vi "Interface.vi"() -> ()   [LabVIEW 2016, in "Operation Interface.lvclass"]
uses:
  Operation Interface.lvclass
  Robot/Universal Robot/Universal Robot.lvclass
  C:/_Code/Development/URLabVIEWInterface/Classes/Application/Application Interfaces/Application Interface/Application Interface.lvclass
  Operation Interface.lvclass/Operation Interface.ctl
  Application Interface/FGVAction.ctl
  Application.lvclass
  Application Interface/Application Interface.lvclass
panel:
  out "Robot Mode":string
  out "robotModeColor":u32(colorbox)
  out "Operational Mode":string
  in  "powerOn":bool
  in  "brakeRelease":bool
  out "Safety Status":string
  out "safetyStatusColor":u32(colorbox)
  in  "restartSafety":bool
  in  "unlockProtectiveStop":bool
  in  "shutdownRobot":bool
  in  "sample rate (ms)":i32
  in  "interface":refnum<class "Operation Interface.lvclass">
  in  "robot":refnum<class "Universal Robot.lvclass">
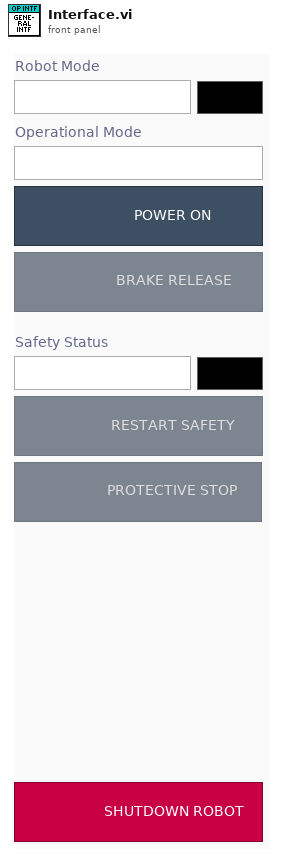
[diagram p1: front panel]
types:
  T1 = typedef "Universal Robot.lvclass/RobotStatus.ctl" = cluster{"Robot Mode":T2, "Operational Mode":T3, "Safety Status":T4, "Remote Control":bool}
  T2 = typedef "Universal Robot.lvclass/RobotMode.ctl" = enum16{"INVALID", "NO_CONTROLLER", "DISCONNECTED", "CONFIRM_SAFETY", "BOOTING", "POWER_OFF", "POWER_ON", "IDLE", "BACKDRIVE", "RUNNING"}
  T3 = typedef "Universal Robot.lvclass/OperationalMode.ctl" = enum16{"NONE", "MANUAL", "AUTOMATIC"}
  T4 = typedef "Universal Robot.lvclass/SafetyStatus.ctl" = enum16{"INVALID", "NORMAL", "REDUCED", "PROTECTIVE_STOP", "RECOVERY", "SAFEGUARD_STOP", "SYSTEM_EMERGENCY_STOP", "ROBOT_EMERGENCY_STOP", "VIOLATION", "FAULT", "AUTOMATIC_MODE_SAFEGAURD_STOP", "SYSTEM_THREE_POSITION_ENABLING_STOP"}
  T5 = typedef "Application Interface.lvclass/FGVAction.ctl" = enum16{"Initialize", "Get Last Status", "Update Status"}
  T6 = typedef "Application.lvclass/FrontPanelControls.ctl" = cluster{"Operation Interface":refnum<vi>, "Program Interface":refnum<vi>, "Command Interface":refnum<vi>, "Socket Interface":refnum<vi>}
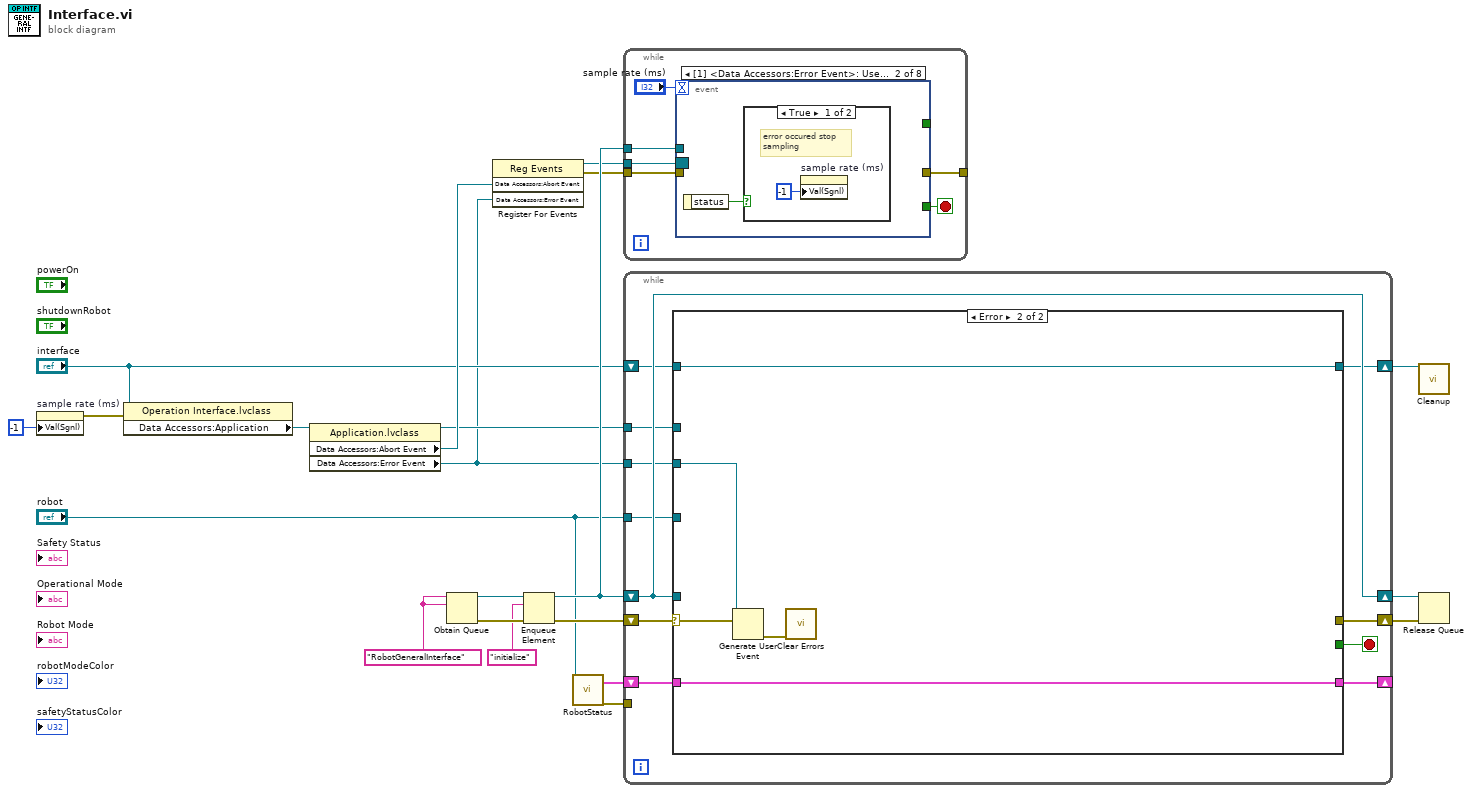
[diagram p0: block diagram]
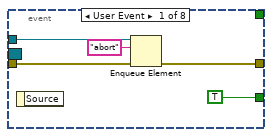
[diagram p2: hidden frame]
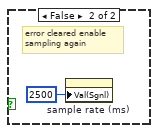
[diagram p3: hidden frame]
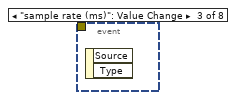
[diagram p4: hidden frame]
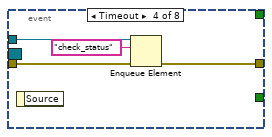
[diagram p5: hidden frame]
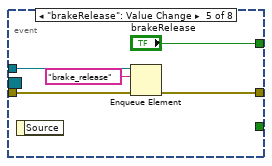
[diagram p6: hidden frame]
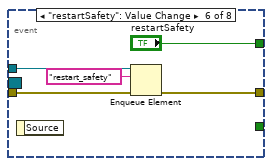
[diagram p7: hidden frame]
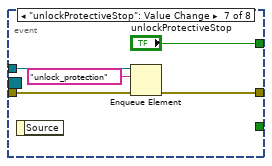
[diagram p8: hidden frame]
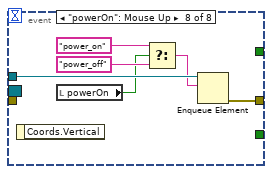
[diagram p9: hidden frame]
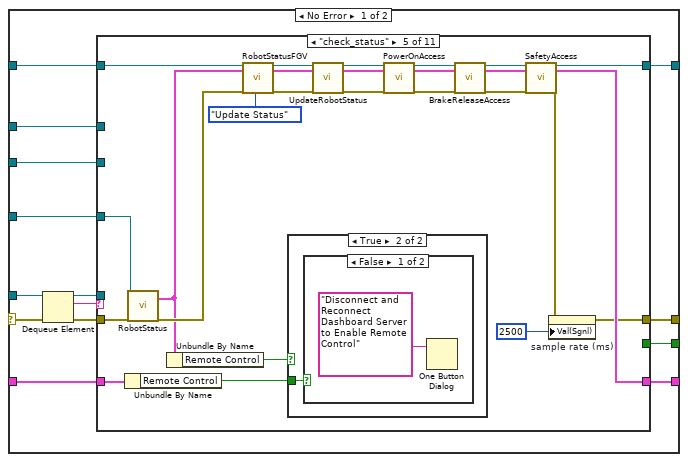
[diagram p10: hidden frame]
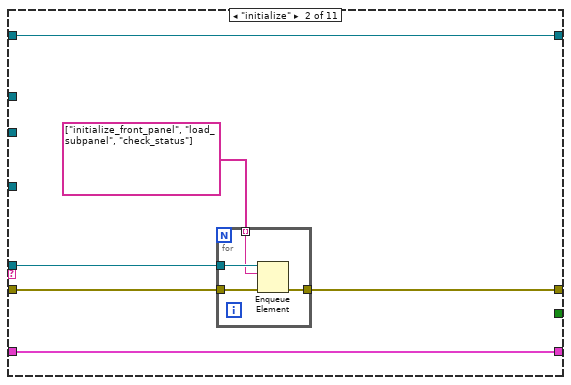
[diagram p12: hidden frame]
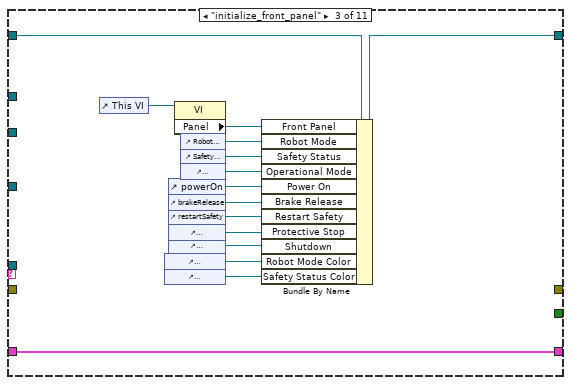
[diagram p13: hidden frame]
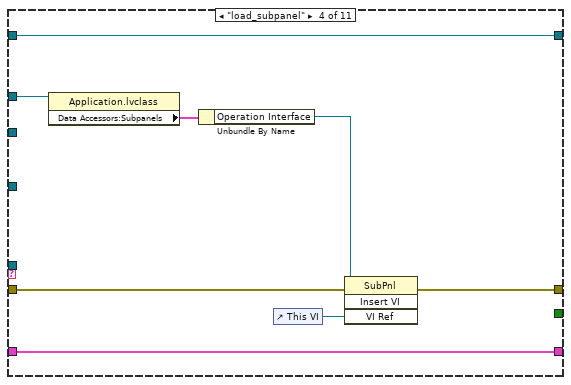
[diagram p14: hidden frame]
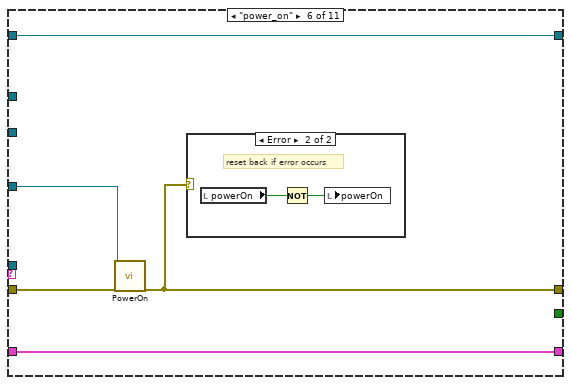
[diagram p17: hidden frame]
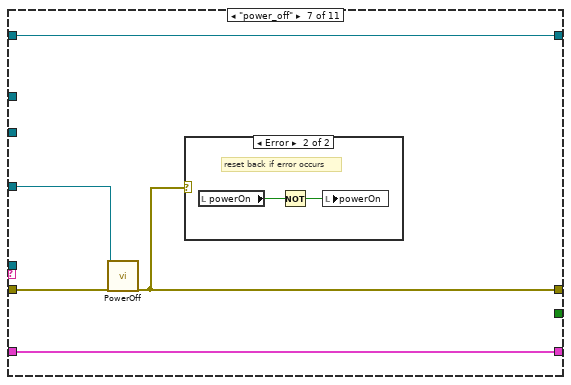
[diagram p19: hidden frame]
diagram:
  w16 = "RobotGeneralInterface" ("name (unnamed)")
  n1 = property on="sample rate (ms)" class="DigNum (strict)"("Val(Sgnl)"=-1 ("Value (Signaling)")) -> (error out=w4:errorcluster)  [unwired: 2 in, 1 out]
  n2 = property class="Operation Interface.lvclass"(reference="interface", error in=w4) -> ("Data Accessors:Application"=w11:refnum<class "Application.lvclass">)  [unwired: 2 out]
  n3 = property class="Application.lvclass"(reference=w11) -> (reference out=w9:refnum<class "Application.lvclass">, "Data Accessors:Abort Event"=w10:refnum<user-event>, "Data Accessors:Error Event"=w6:refnum<user-event>)  [unwired: 1 in, 1 out]
  n4 = Obtain Queue(name (unnamed)=w16, element data type=w16) -> (queue out=w20:refnum<queue>, error out=w21:errorcluster)  [unwired: 3 in, 1 out]
  n5 = register-events(w10, w6) -> (reference out=w12:refnum<event-registration>, error out=w13:errorcluster)  [unwired: 2 in]
  n6 = Enqueue Element(queue=w20, element="initialize", error in (no error)=w21) -> (queue out=w17:refnum<queue>, error out=w18:errorcluster)  [unwired: 1 in, 1 out]
  n7 = call-dynamic "RobotStatus.vi"("Universal Robot.lvclass in"="robot") -> ("Robot Status"=w2:T1, "error out"=w1:errorcluster)  [unwired: 16 in, 1 out]
  n8 = while {
    tunnel: w17 -> [w27]
    tunnel: w13 -> [w26]
    tunnel: w12 -> [w25]
    tunnel: [w24] -> _
    stop <- w23 stop-if-true
    n9 = event shown="[1] <Data Accessors:Error Event>: User Event" {
      selector: w25 -> [_ _ _ _ _ _ _ _]
      dyn-events: _ -> [_ _ _ _ _ _ _ _]
      timeout: "sample rate (ms)" -> [_ _ _ _ _ _ _ _]
      tunnel: w27 -> [w32 _ _ w39 w44 w49 w54 w60]
      tunnel: w26 -> [w31 _ _ w38 w43 w48 w53 _]
      tunnel: [w30 _ _ w37 w42 w47 w52 w59] -> w24
      tunnel: [TRUE _ _ _ _ _ _ _] -> w23
      tunnel: [_ _ _ _ "brakeRelease" "restartSafety" "unlockProtectiveStop" _] -> _
      event User Event {
        n10 = event-data() -> ()  [unwired: 1 in, 1 out]
        n11 = Enqueue Element(queue=w32, element="abort", error in (no error)=w31) -> (error out=w30:errorcluster)  [unwired: 1 in, 2 out]
      }
      event User Event {
        n12 = event-data() -> ("status"=w33:bool)  [unwired: 1 in]
        n13 = case shown="True" w33 {
          frame True {
            # "error occured stop\nsampling"
            n14 = property on="sample rate (ms)" class="DigNum (strict)"("Val(Sgnl)"=-1 ("Value (Signaling)")) -> ()  [unwired: 2 in, 2 out]
          }
          frame False {
            # "error cleared enable\nsampling again"
            n15 = property on="sample rate (ms)" class="DigNum (strict)"("Val(Sgnl)"=2500 ("Value (Signaling)")) -> ()  [unwired: 2 in, 2 out]
          }
        }
      }
      event "sample rate (ms)": Value Change {
        n16 = event-data() -> ()  [unwired: 1 in, 2 out]
      }
      event Timeout {
        n17 = event-data() -> ()  [unwired: 1 in, 1 out]
        n18 = Enqueue Element(queue=w39, element="check_status", error in (no error)=w38) -> (error out=w37:errorcluster)  [unwired: 1 in, 2 out]
      }
      event "brakeRelease": Value Change {
        n19 = event-data() -> ()  [unwired: 1 in, 1 out]
        n20 = Enqueue Element(queue=w44, element="brake_release", error in (no error)=w43) -> (error out=w42:errorcluster)  [unwired: 1 in, 2 out]
      }
      event "restartSafety": Value Change {
        n21 = event-data() -> ()  [unwired: 1 in, 1 out]
        n22 = Enqueue Element(queue=w49, element="restart_safety", error in (no error)=w48) -> (error out=w47:errorcluster)  [unwired: 1 in, 2 out]
      }
      event "unlockProtectiveStop": Value Change {
        n23 = event-data() -> ()  [unwired: 1 in, 1 out]
        n24 = Enqueue Element(queue=w54, element="unlock_protection", error in (no error)=w53) -> (error out=w52:errorcluster)  [unwired: 1 in, 2 out]
      }
      event "powerOn": Mouse Up {
        n25 = event-data() -> ()  [unwired: 1 in, 1 out]
        n26 = local read "powerOn"() -> (w55:bool)
        n27 = Select(t="power_on", s=w55, f="power_off") -> (s? t:f=w57:string)
        n28 = Enqueue Element(queue=w60, element=w57) -> (error out=w59:errorcluster)  [unwired: 2 in, 2 out]
      }
    }
  }
  n29 = while {
    shift-right: [w69] -> w14
    shift-left: w18 -> [w71]
    shift-right: [w70] -> w15
    shift-left: w17 -> [w70]
    tunnel: "robot" -> [w66]
    tunnel: w6 -> [w65]
    tunnel: w9 -> [w64]
    shift-right: [w63] -> w7
    shift-left: "interface" -> [w67]
    shift-right: [w62] -> _
    shift-left: w2 -> [w61]
    tunnel: w1 -> [_]
    stop <- w68 stop-if-true
    n30 = case shown="Error" w71 {
      selector: w71 -> [w84 w189]
      tunnel: w70 -> [w85 _]
      tunnel: [w80 _] -> w69
      tunnel: [w79 _] -> w68
      tunnel: w67 -> [w78 w188]
      tunnel: w66 -> [w77 _]
      tunnel: w65 -> [w76 w190]
      tunnel: w64 -> [w75 _]
      tunnel: [w74 w188] -> w63
      tunnel: [w73 w187] -> w62
      tunnel: w61 -> [w72 w187]
      frame No Error {
        n31 = Dequeue Element(queue=w85, error in (no error)=w84) -> (queue out=w81:refnum<queue>, element=w82:string, error out=w83:errorcluster)  [unwired: 1 in, 1 out]
        n32 = case shown="\"check_status\"" w82 {
          tunnel: w83 -> [w88 w92 _ w117 w146 w152 w159 w166 w171 w176 w183]
          tunnel: w81 -> [_ w93 _ _ _ _ _ _ _ _ _]
          tunnel: [w88 w91 _ w121 w122 w150 w157 w164 w169 w174 w182] -> w80
          tunnel: [_ _ _ _ _ _ _ _ _ _ TRUE] -> w79
          tunnel: w78 -> [w87 w94 w113 w119 w137 w151 w160 w167 w172 w177 w184]
          tunnel: w77 -> [_ _ _ _ w145 w153 w158 w165 w170 w175 _]
          tunnel: w76 -> [_ _ _ _ _ _ _ _ _ _ _]
          tunnel: w75 -> [_ _ _ w118 _ _ _ _ _ _ w181]
          tunnel: [w87 w94 w112 w119 w131 w151 w160 w167 w172 w177 w184] -> w74
          tunnel: [w86 w89 w99 w114 w125 w149 w156 w163 w168 w173 w178] -> w73
          tunnel: w72 -> [w86 w89 w99 w114 w128 w149 w156 w163 w168 w173 w178]
          frame Default {
          }
          frame "initialize" {
            n33 = for {
              tunnel: w93 -> [w98]
              tunnel: w92 -> [w97]
              tunnel: [w96] -> w91
              tunnel: string[] ["initialize_front_panel", "load_subpanel", "check_status"] -> [w95] mode=indexing
              n34 = Enqueue Element(queue=w98, element=w95, error in (no error)=w97) -> (error out=w96:errorcluster)  [unwired: 1 in, 2 out]
            }
          }
          frame "initialize_front_panel" {
            n35 = control-ref of="This VI"() -> (w102:refnum<vi>)
            n36 = control-ref of="robotModeColor"() -> (w110:refnum<vi>)
            n37 = control-ref of="safetyStatusColor"() -> (w103:refnum<vi>)
            n38 = control-ref of="powerOn"() -> (w108:refnum<vi>)
            n39 = control-ref of="brakeRelease"() -> (w107:refnum<vi>)
            n40 = control-ref of="restartSafety"() -> (w106:refnum<vi>)
            n41 = control-ref of="unlockProtectiveStop"() -> (w105:refnum<vi>)
            n42 = control-ref of="shutdownRobot"() -> (w104:refnum<vi>)
            n43 = property class="VI"(reference=w102) -> ("Panel"=w101:refnum<vi>)  [unwired: 1 in, 2 out]
            n44 = control-ref of="Robot Mode"() -> (w111:refnum<vi>)
            n45 = control-ref of="Safety Status"() -> (w100:refnum<vi>)
            n46 = control-ref of="Operational Mode"() -> (w109:refnum<vi>)
            n47 = Bundle By Name(cluster=w113, "Front Panel"=w101, "Robot Mode"=w111, "Safety Status"=w100, "Operational Mode"=w109, "Power On"=w108, "Brake Release"=w107, "Restart Safety"=w106, "Protective Stop"=w105, "Shutdown"=w104, "Robot Mode Color"=w110, "Safety Status Color"=w103) -> (w112:refnum<class "Operation Interface.lvclass">)
          }
          frame "load_subpanel" {
            n48 = property class="Application.lvclass"(reference=w118) -> ("Data Accessors:Subpanels"=w116:T6)  [unwired: 1 in, 2 out]
            n49 = Unbundle By Name(w116) -> ("Operation Interface"=w115:refnum<vi>)
            n50 = control-ref of="This VI"() -> (w120:refnum<vi>)
            n51 = invoke class="SubPnl" method="Insert VI"(reference=w115, error in=w117, "VI Ref"=w120) -> (error out=w121:errorcluster)  [unwired: 1 in, 3 out]
          }
          frame "check_status" {
            n52 = Unbundle By Name(w128) -> ("Remote Control"=w123:bool)
            n53 = call-dynamic "RobotStatus.vi"("Universal Robot.lvclass in"=w145, "error in (no error)"=w146) -> ("Robot Status"=w127:T1, "error out"=w144:errorcluster)  [unwired: 15 in, 1 out]
            n54 = Unbundle By Name(w127) -> ("Remote Control"=w124:bool)
            n55 = call "RobotStatusFGV.vi"("Application Interface in"=w137, "Robot Status in"=w127, "Action (Read)"=FGVAction."Update Status") -> ("Application Interface out"=w136:refnum<class "Operation Interface.lvclass">, "Robot Status out"=w126:T1)  [unwired: 14 in, 1 out]
            n56 = case shown="True" w124 {
              tunnel: w123 -> [_ w147]
              frame False {
              }
              frame True {
                n57 = case shown="False" w147 {
                  frame False {
                    n58 = One Button Dialog(message="Disconnect and Reconnect Dashboard Server to Enable Remote Control") -> ()  [unwired: 1 in, 1 out]
                  }
                  frame True {
                  }
                }
              }
            }
            n59 = call "UpdateRobotStatus.vi"("Operation Interface in"=w136, "Robot Status"=w126, "error in (no error)"=w144) -> ("Operation Interface out"=w143:refnum<class "Operation Interface.lvclass">, "Robot Status Out"=w142:T1, "error out"=w141:errorcluster)  [unwired: 14 in]
            n60 = call "PowerOnAccess.vi"("Operation Interface in"=w143, "Robot Status"=w142, "error in (no error)"=w141) -> ("Operation Interface out"=w140:refnum<class "Operation Interface.lvclass">, "Robot Status Out"=w138:T1, "error out"=w139:errorcluster)  [unwired: 14 in]
            n61 = call "BrakeReleaseAccess.vi"("Operation Interface in"=w140, "Robot Status in"=w138, "error in (no error)"=w139) -> ("Operation Interface out"=w134:refnum<class "Operation Interface.lvclass">, "Robot Status out"=w132:T1, "error out"=w133:errorcluster)  [unwired: 14 in]
            n62 = call "SafetyAccess.vi"("Operation Interface in"=w134, "Robot Status In"=w132, "error in (no error)"=w133) -> ("Operation Interface out"=w131:refnum<class "Operation Interface.lvclass">, "Robot Status Out"=w125:T1, "error out"=w129:errorcluster)  [unwired: 14 in]
            n63 = property on="sample rate (ms)" class="DigNum (strict)"(error in=w129, "Val(Sgnl)"=2500 ("Value (Signaling)")) -> (error out=w122:errorcluster)  [unwired: 1 in, 1 out]
          }
          frame "power_on" {
            n64 = call-dynamic "PowerOn.vi"("Universal Robot.lvclass in"=w153, "error in (no error)"=w152) -> ("error out"=w150:errorcluster)  [unwired: 16 in, 1 out]
            n65 = case shown="Error" w150 {
              frame No Error {
              }
              frame Error {
                # "reset back if error occurs"
                n66 = local read "powerOn"() -> (w155:bool)
                n67 = Not(x=w155) -> (.not. x?=w154:bool)
                n68 = local write "powerOn"(w154) -> ()
              }
            }
          }
          frame "power_off" {
            n69 = call-dynamic "PowerOff.vi"("Universal Robot.lvclass in"=w158, "error in (no error)"=w159) -> ("error out"=w157:errorcluster)  [unwired: 16 in, 1 out]
            n70 = case shown="Error" w157 {
              frame No Error {
              }
              frame Error {
                # "reset back if error occurs"
                n71 = local read "powerOn"() -> (w162:bool)
                n72 = Not(x=w162) -> (.not. x?=w161:bool)
                n73 = local write "powerOn"(w161) -> ()
              }
            }
          }
          frame "brake_release" {
            n74 = call-dynamic "BrakeRelease.vi"("Universal Robot.lvclass in"=w165, "error in (no error)"=w166) -> ("error out"=w164:errorcluster)  [unwired: 16 in, 1 out]
          }
          frame "restart_safety" {
            n75 = call-dynamic "RestartSafety.vi"("Universal Robot.lvclass in"=w170, "error in (no error)"=w171) -> ("error out"=w169:errorcluster)  [unwired: 16 in, 1 out]
          }
          frame "unlock_protection" {
            n76 = call-dynamic "UnlockProtectiveStop.vi"("Universal Robot.lvclass in"=w175, "error in (no error)"=w176) -> ("error out"=w174:errorcluster)  [unwired: 16 in, 1 out]
          }
          frame "abort" {
            n77 = property class="Application.lvclass"(reference=w181) -> ("Data Accessors:Subpanels"=w180:T6)  [unwired: 1 in, 2 out]
            n78 = Unbundle By Name(w180) -> ("Operation Interface"=w179:refnum<vi>)
            n79 = invoke class="SubPnl" method="Remove VI"(reference=w179, error in=w183) -> (error out=w182:errorcluster)  [unwired: 1 in, 2 out]
          }
        }
      }
      frame Error {
        n80 = Generate User Event(user event=w190, event data cluster=w189) -> (error out=w186:errorcluster)  [unwired: 2 in, 1 out]
        n81 = call <vilib>:"Clear Errors.vi"("error in (no error)"=w186) -> ()  [unwired: 5 in, 2 out]
      }
    }
  }
  n82 = call "Cleanup.vi"("Operation Interface in"=w7) -> ()  [unwired: 19 in]
  n83 = Release Queue(queue=w15, error in (no error)=w14) -> ()  [unwired: 1 in, 3 out]
